vi "taskWithWrongConnectorPane.vi"(11 "ITask in":refnum<class "ITask.lvclass">) -> (3 "ITask out":refnum<class "ITask.lvclass">)   [LabVIEW 2023, in "TaskMock.lvclass"]
uses:
  TaskMock.lvclass
  TaskMock.lvclass/TaskMock.ctl
  source/ITask/ITask.lvclass
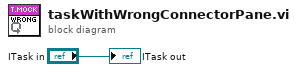
[diagram p0: block diagram]
diagram:
  "ITask out" <- "ITask in"
